vi "Flang Controller.vi"(8 "error in":errorcluster) -> ()   [LabVIEW 2019]
doc: "This VI executes continuously carrying out the current operation and responding to updates or new operations. It will often contain the timing or control code that is difficult to place directly in TeleOp. This VI generally opens all sensors and motors and isolates the rest of the robot code from knowing how the operations are carried out."
uses:
  <vilib>/Rock Robotics/WPI/Framework/Completion Status.ctl
  Flang Setpoints.ctl
  Flang Operations.ctl
  <vilib>/Rock Robotics/WPI/ThirdParty/Phoenix-LabVIEW/Motor Controller/Controls/CTRE_Phoenix_MotorControl_NeutralMode.ctl
  <vilib>/Rock Robotics/WPI/ThirdParty/Phoenix-LabVIEW/Motor Controller/Controls/CTRE_Phoenix_MotorControl_ControlMode.ctl
  Framework/Robot Global Data.vi
  <vilib>/Rock Robotics/Network Tables/NT Write Boolean.vi
panel:
  in  "Interactive Values":T1
  out "Current\nCmd":string
  in  "Buttons":cluster{"Execute Cmd":bool, "Abort Cmd":bool}
  out "Command Timing":cluster{"Start Time (ms)":u32, "Iterations":i32}
  out "Status":T3
  # "Tip: It may be helpful to observe inputs and sensor values.\nYou may also want to display tuning or debugging controls."
  # "Interactive Command: You may fill in the settings for a command\nand schedule it with the Execute button. You can observe and abort\nany command while fine tuning the code for the controller."
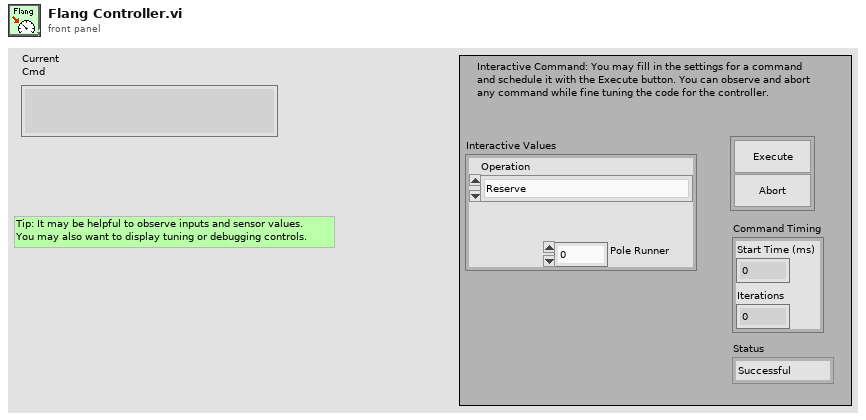
[diagram p1: front panel]
types:
  T1 = typedef "Flang Setpoints.ctl" = cluster{"Operation":T2, "Pole Runner":dbl}
  T2 = typedef "Flang Operations.ctl" = enum16{"Reserve", "Read Current", "Immediate"}
  T3 = typedef "Completion Status.ctl" = enum16{"Successful", "Aborted", "Incomplete"}
  T4 = typedef "CTRE_Phoenix_MotorControl_NeutralMode.ctl" = enum8{"EEPROMSetting", "Override to Coast", "Override to Brake"}
  T5 = typedef "WPI_MotorControlDeviceRef.ctl" = cluster{"DeviceStatus":errorcluster, "Type":T6, "PWM":cluster{"PWM Channel":T7, "DeadBand":T8}, "CAN":cluster{"Device Number":u8, "SetOutput VI Ref":variant, "GetOutput VI Ref":variant, "Enable VI Ref":variant, "Disable VI Ref":variant, "Data":variant}, "Invert":bool, "DIO PWM":cluster{"PWM \"Enable\" Channel":T7, "DIOChannel":T9, "PWM Rate":dbl}}
  T6 = typedef "WPI_MotorControlType.ctl" = enum16{"PWM", "CAN", "DIO PWM"}
  T7 = typedef "FPGA_DIOPWMChannel.ctl" = enum8{"PWM 0", "PWM 1", "PWM 2", "PWM 3", "PWM 4", "PWM 5", "PWM 6", "PWM 7", "PWM 8", "PWM 9", "PWM MXP 0", "PWM MXP 1", "PWM MXP 2", "PWM MXP 3", "PWM MXP 4", "PWM MXP 5", "PWM MXP 6", "PWM MXP 7", "PWM MXP 8", "PWM MXP 9", "Invalid"}
  T8 = typedef "WPI_PWMDeadband.ctl" = cluster{"Name":string, "maxPositivePwm":i32, "minPositivePwm":i32, "centerPwm":i32, "maxNegativePwm":i32, "minNegativePwm":i32, "angularRange":u16}
  T9 = typedef "FPGA_DIOChannel.ctl" = enum8{"DIO 0", "DIO 1", "DIO 2", "DIO 3", "DIO 4", "DIO 5", "DIO 6", "DIO 7", "DIO 8", "DIO 9", "DIO MXP 0", "DIO MXP 1", "DIO MXP 2", "DIO MXP 3", "DIO MXP 4", "DIO MXP 5", "DIO MXP 6", "DIO MXP 7", "DIO MXP 8", "DIO MXP 9", "DIO MXP 10", "DIO MXP 11", "DIO MXP 12", "DIO MXP 13", "DIO MXP 14", "DIO MXP 15", "SPI Port CS1", "SPI Port CS2", "SPI Port CS3", "SPI Port MISO", "SPI Port MOSI", "Invalid"}
  T10 = typedef "Command Status Info.ctl" = cluster{"Name":string, "Status":T3, "notifier out":T11}
  T11 = typedef "Completion Notifier.ctl" = refnum<notifier>
  T12 = cluster{"Current Command":T1, "Command Timing":cluster{"Start Time (ms)":u32, "Iterations":i32}, "Command Arguments":cluster{"Command Info":T10, "Description":string, "Default Command":T1, "queue out":refnum<queue>, "Subsystem Name":string}}
  T13 = typedef "CTRE_Phoenix_MotorControl_ControlMode.ctl" = u16
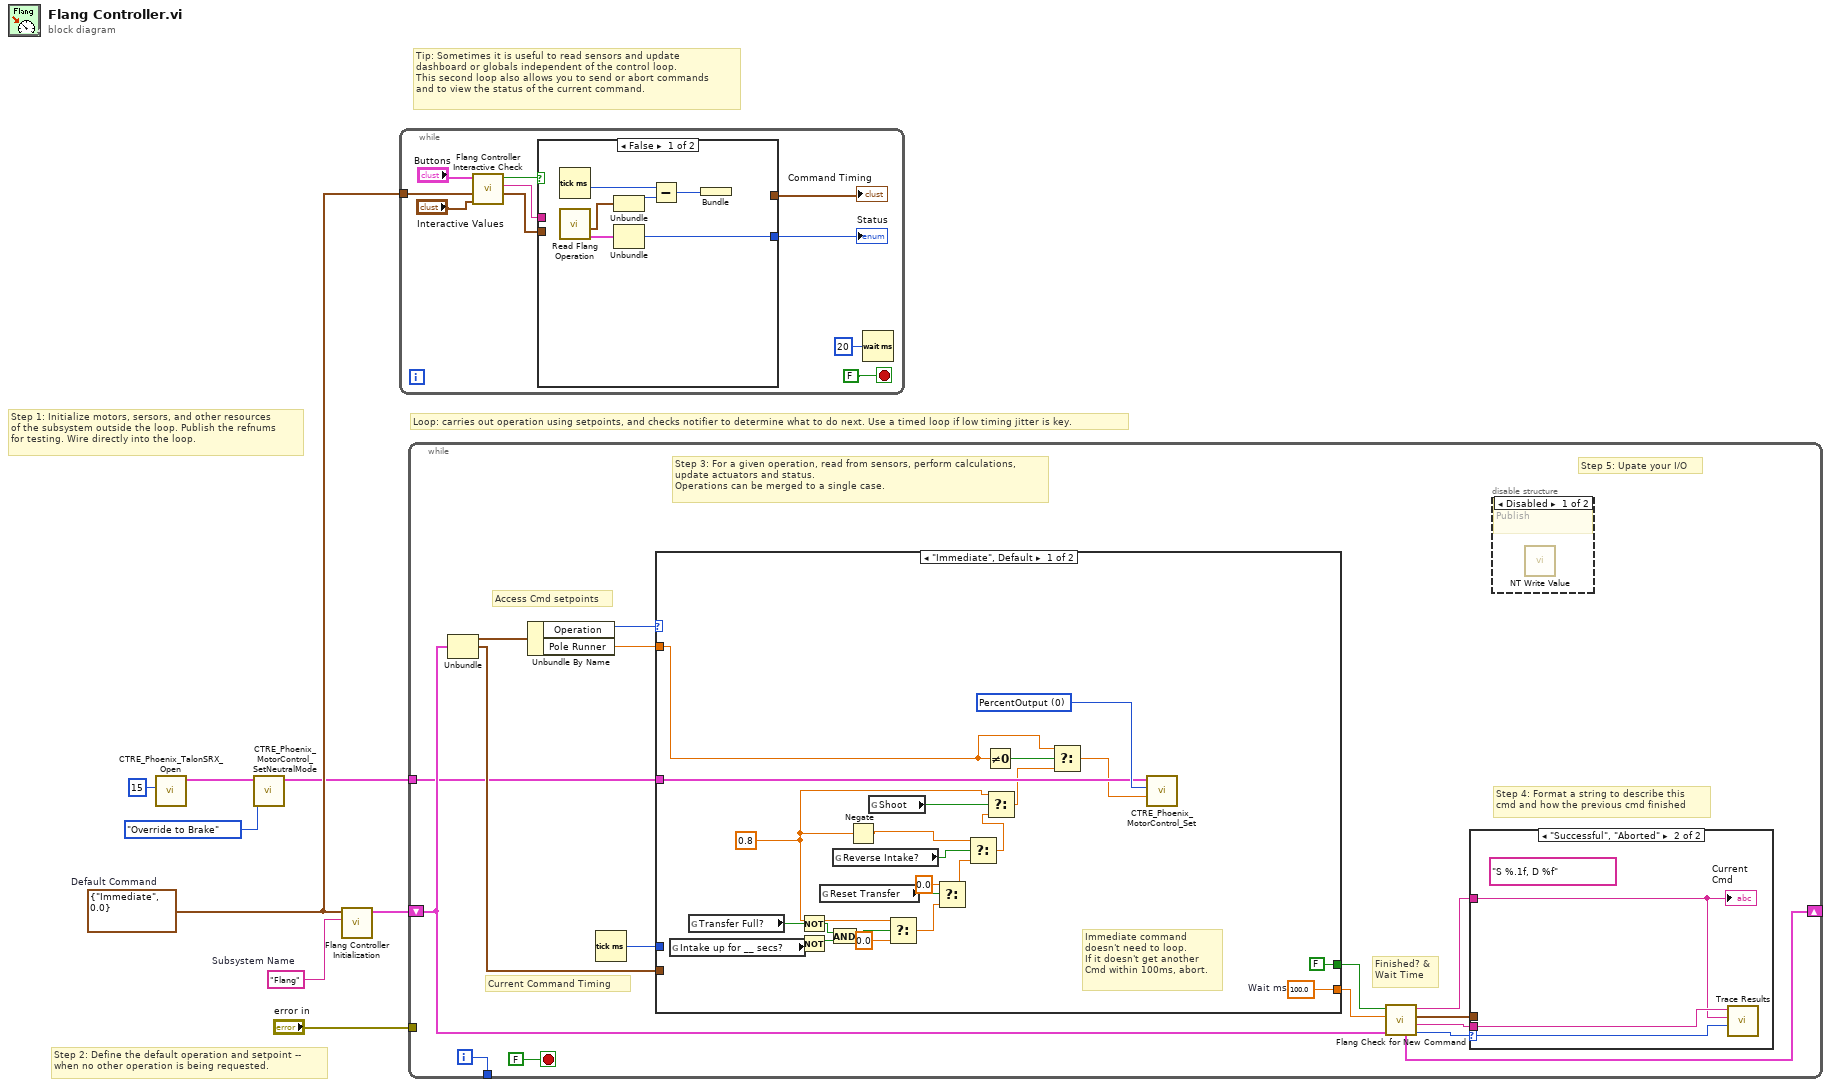
[diagram p0: block diagram]
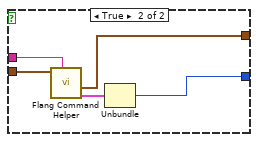
[diagram p2: hidden frame]
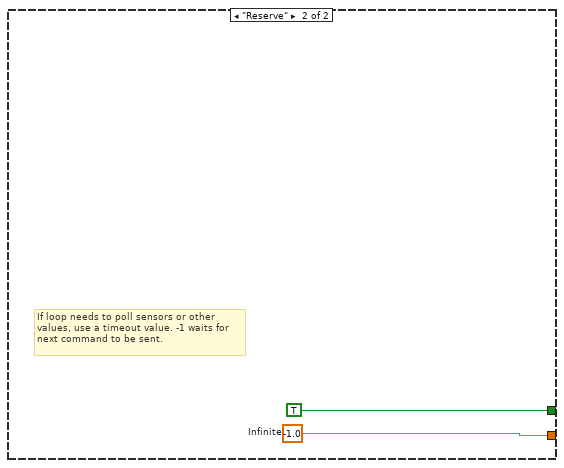
[diagram p5: hidden frame]
diagram:
  w5 = T1 {"Operation"=enum."Immediate", "Pole Runner"=0.0}  # Default Command
  w6 = "Flang"  # Subsystem Name
  # "Tip: Sometimes it is useful to read sensors and update\ndashboard or globals independent of the control loop.\nThis second loop also allows you to send or abort commands\nand to view the status of the current command."
  # "Step 2: Define the default operation and setpoint --\nwhen no other operation is being requested."
  # "Step 1: Initialize motors, sersors, and other resources\nof the subsystem outside the loop. Publish the refnums\nfor testing. Wire directly into the loop."
  # "Loop: carries out operation using setpoints, and checks notifier to determine what to do next. Use a timed loop if low timing jitter is key."
  n1 = call <vilib>:"CTRE_Phoenix_TalonSRX_Open.vi"("Device Number"=u8 15) -> ("CAN Talon SRX Ref"=w3:T5)  [unwired: 9 in, 1 out]
  n2 = call <vilib>:"CTRE_Phoenix_MotorControl_SetNeutralMode.vi"("Motor Control Neutral Mode"=CTRE_Phoenix_MotorControl_NeutralMode."Override to Brake", "PhoenixMotorControlDevRef"=w3) -> ("PhoenixMotorControlDevRef"=w2:T5)  [unwired: 8 in, 1 out]
  n3 = call "Flang Controller Initialization.vi"("Subsystem Name"=w6, "Default Command"=w5) -> ("Current Command"=w7:T12)  [unwired: 9 in]
  n4 = while {
    tunnel: w5 -> [w15]
    stop <- FALSE stop-if-true
    n5 = call "Flang Controller Interactive Check.vi"("Interactive Command in"="Interactive Values", "Default Command"=w15, "Buttons"="Buttons") -> ("Interactive Command out"=w12:T1, "Trace String"=w13:string, "Schedule"=w14:bool)  [unwired: 6 in]
    n6 = case shown="False" w14 {
      tunnel: [w24 w29] -> w11
      tunnel: w12 -> [_ w27]
      tunnel: [_ w25] -> w10
      tunnel: w13 -> [_ w28]
      frame False {
        n7 = Tick Count (ms)() -> (millisecond timer value=w21:u32)
        n8 = call "Read Flang Operation.vi"() -> ("Command Info"=w19:T10, "SubSystem Data"=w20:T1)  [unwired: 9 in, 1 out]
        n9 = Unbundle(w20) -> ("Operation"=w23:T2)  [unwired: 1 out]
        n10 = Unbundle(w19) -> ("Status"=w24:T3)  [unwired: 2 out]
        n11 = Subtract(x=w21, y=w23) -> (x-y=w22:u32)
        n12 = Bundle(w22) -> ()  [unwired: 1 in, 1 out]
      }
      frame True {
        n13 = call "Flang Command Helper.vi"("Description"=w28, "SubSystem Data"=w27) -> ("Command Info Out"=w26:T10, "Command Timing"=w25:cluster{"Start Time (ms)":u32, "Iterations":i32})  [unwired: 7 in, 1 out]
        n14 = Unbundle(w26) -> ("Status"=w29:T3)  [unwired: 2 out]
      }
    }
    "Status" <- w11
    "Command Timing" <- w10
    n15 = Wait (ms)(milliseconds to wait=u32 20) -> ()  [unwired: 1 out]
  }
  n16 = while {
    shift-right: [w39] -> _
    shift-left: w7 -> [w32]
    tunnel: [w44] -> _
    tunnel: "error in" -> [_]
    tunnel: w2 -> [w31]
    i -> [w44]
    stop <- FALSE stop-if-true
    # "Step 5: Upate your I/O"
    # "Step 4: Format a string to describe this\ncmd and how the previous cmd finished"
    # "Current Command Timing"
    # "Access Cmd setpoints"
    # "Finished? &\nWait Time"
    # "Step 3: For a given operation, read from sensors, perform calculations,\nupdate actuators and status.\nOperations can be merged to a single case."
    n17 = Unbundle(w32) -> ("Current Command"=w43:T1, "Command Timing"=w40:cluster{"Start Time (ms)":u32, "Iterations":i32})  [unwired: 1 out]
    n18 = Unbundle By Name(w43) -> ("Operation"=w42:T2, "Pole Runner"=w30:dbl)
    n19 = Tick Count (ms)() -> (millisecond timer value=w41:u32)
    n20 = case shown="\"Immediate\", Default" w42 {
      tunnel: [w71 w73] -> w37
      tunnel: [FALSE ("ignore previous (F)") TRUE ("ignore previous (F)")] -> w38
      tunnel: w40 -> [_ _]
      tunnel: w41 -> [_ _]
      tunnel: w31 -> [w60 _]
      tunnel: w30 -> [w57 _]
      frame "Immediate", Default {
        w49 = 0.8 ("t")
        w70 = T13 0 items=["PercentOutput"=0, "Position"=1, "Velocity"=2, "Current"=3, "Follower"=5, "MotionProfile"=6, "MotionMagic"=7, "MotionProfileArc"=10, "Disabled"=15] ("Control Mode")
        w71 = 100.0  # Wait ms
        # "Immediate command\ndoesn't need to loop.\nIf it doesn't get another\nCmd within 100ms, abort."
        n21 = global read "Robot Global Data.vi" "Intake up for __ secs?"() -> (w66:bool)
        n22 = global read "Robot Global Data.vi" "Transfer Full?"() -> (w65:bool)
        n23 = Not(x=w65) -> (.not. x?=w62:bool)
        n24 = Not(x=w66) -> (.not. x?=w61:bool)
        n25 = global read "Robot Global Data.vi" "Reset Transfer"() -> (w68:bool)
        n26 = And(x=w62, y=w61) -> (x .and. y?=w64:bool)
        n27 = global read "Robot Global Data.vi" "Reverse Intake?"() -> (w51:bool)
        n28 = Negate(x=w49) -> (-x=w50:dbl)
        n29 = global read "Robot Global Data.vi" "Shoot"() -> (w69:bool)
        n30 = Select(t=w49, s=w64, f=0.0) -> (s? t:f=w63:dbl)
        n31 = Select(t=0.0, s=w68, f=w63) -> (s? t:f=w53:dbl)
        n32 = Select(t=w50, s=w51, f=w53) -> (s? t:f=w52:dbl)
        n33 = Not Equal To 0?(x=w57) -> (x != 0?=w58:bool)
        n34 = Select(t=w49, s=w69, f=w52) -> (s? t:f=w56:dbl)
        n35 = Select(t=w57, s=w58, f=w56) -> (s? t:f=w55:dbl)
        n36 = call <vilib>:"CTRE_Phoenix_MotorControl_Set.vi"("Output"=w55, "Control Mode"=w70, "PhoenixMotorControlDevRef"=w60) -> ()  [unwired: 7 in, 2 out]
      }
      frame "Reserve" {
        w73 = -1.0  # Infinite
        # "If loop needs to poll sensors or other\nvalues, use a timeout value. -1 waits for\nnext command to be sent."
      }
    }
    n37 = call "Flang Check for New Command.vi"("Current Command"=w32, "Wait time (ms)"=w37, "Finished?"=w38) -> ("Completion"=w33:T3, "Subsystem Name"=w34:string, "Current Command"=w35:T1, "Initial Trace String"=w36:string, "NextCommand"=w39:T12)  [unwired: 4 in]
    n38 = case shown="\"Successful\", \"Aborted\"" w33 {
      selector: w33 -> [_ w48]
      tunnel: w36 -> [_ w46]
      tunnel: w35 -> [_ _]
      tunnel: w34 -> [_ w47]
      frame "Incomplete", Default {
        # "Continuing current command"
      }
      frame "Successful", "Aborted" {
        (unwired) "S %.1f, D %f" ("format string")
        # "Report and setup for next command"
        n39 = call <vilib>:"Trace Results.vi"("Status of previous command"=w48, "Description"=w46, "Subsystem"=w47) -> ()  [unwired: 9 in]
        "Current\nCmd" <- w46
      }
    }
    n40 = disable-structure shown="Disabled" {
      frame Disabled {
        # "Publish"
        n41 = call-poly <vilib>:"NT Write Value.vi"() -> ()  [unwired: 11 in, 1 out]
      }
      frame Enabled {
      }
    }
  }
